vi "Configure test.vi"(6 "Assert VI Path":path, 7 "Existing Queue Elements":string, 8 "error in (no error)":errorcluster, 11 "Basic Integer in":refnum<class "Integer.lvclass">) -> (0 "error out":errorcluster, 3 "Basic Integer out":refnum<class "Integer.lvclass">)   [LabVIEW 2018, in "Integer.lvclass"]
uses:
  Integer.lvclass
  dd54bd95-9200-4918-9d80-7db4f8b1e5ab.vi
  <vilib>/JDP Science/JSONtext/Find Item.vi
  dd54bd95-9200-4918-9d80-7db4f8b1e5ab.vi/2536fbfc-b4f4-4be9-af8d-f468e540d464.vi
  dd54bd95-9200-4918-9d80-7db4f8b1e5ab.vi/6bdf9347-2671-4b8c-90fa-16a3674c5fbd.vi
  <vilib>/JDP Science/JSONtext/String Subset.vi
  Test Class String IDs.vi
  <vilib>/JDP Science/JSONtext/Parsing/Parse Full Path or Item Name.vi
  <vilib>/JDP Science/JSONtext/Offset/Find Item Locations by Path.vi
  <vilib>/JDP Science/JSONtext/JSON text to Variant.vi
  <vilib>/JDP Science/JSONtext/Variant to JSON Text.vi
  <vilib>/JDP Science/JSONtext/Set Item.vi
  Test.lvclass
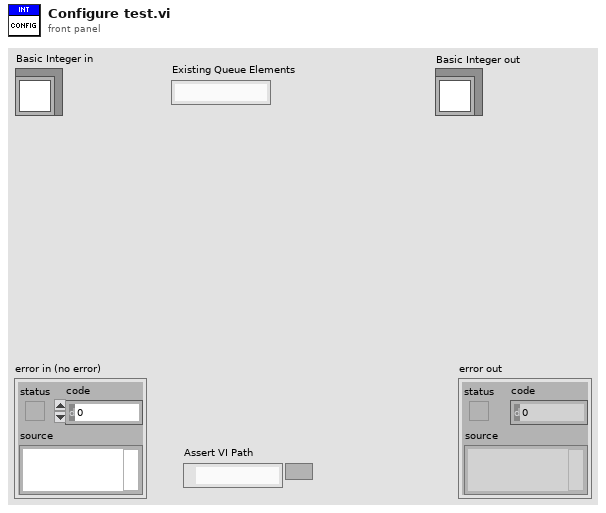
[diagram p1: front panel]
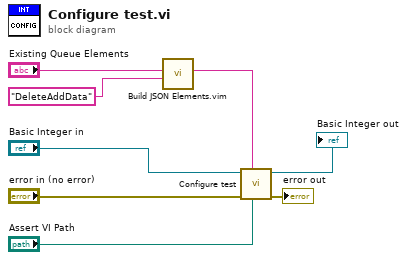
[diagram p0: block diagram]
diagram:
  n1 = call "Build JSON Elements.vim"("Append Element(s)"="DeleteAddData", "JSON Elements in ({})"="Existing Queue Elements") -> ("JSON Elements out"=w4:string)  [unwired: 9 in]
  n2 = call-parent "Configure test.vi"("Assert VI Path"="Assert VI Path", "Existing Queue Elements"=w4, "error in (no error)"="error in (no error)", "Basic Test in"="Basic Integer in") -> ("error out"=→"error out":errorcluster, "Test out"=→"Basic Integer out":refnum<class "Integer.lvclass">)  [unwired: 6 in]
